vi "Read Bus.vi"(8 "error in (no error)":errorcluster, 11 "DigitalGraph.lvclass in":refnum<class "DigitalGraph.lvclass">) -> (0 "error out":errorcluster, 2 "Bus":refnum<vi>, 3 "DigitalGraph.lvclass out":refnum<class "DigitalGraph.lvclass">)   [LabVIEW 2015, in "DigitalGraph.lvclass"]
uses:
  DigitalGraph.lvclass
  DigitalGraph.lvclass/DigitalGraph.ctl
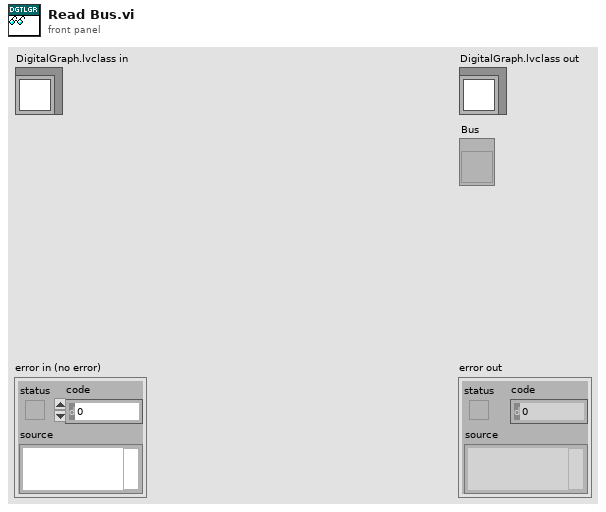
[diagram p1: front panel]
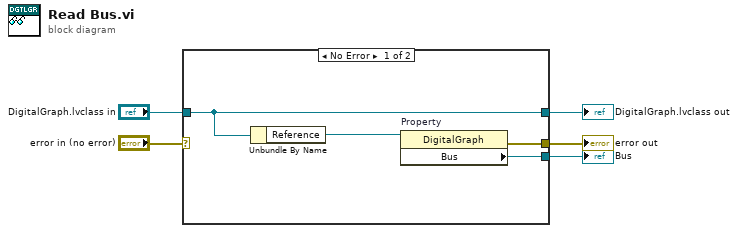
[diagram p0: block diagram]
diagram:
  n1 = case shown="No Error" "error in (no error)" {
    selector: "error in (no error)" -> [_ w11]
    tunnel: [w8 w11] -> w4
    tunnel: [w7 w10] -> w2
    tunnel: "DigitalGraph.lvclass in" -> [w7 w10]
    tunnel: [w9 _] -> w1
    frame No Error {
      n2 = Unbundle By Name(w7) -> ("Reference"=w6:refnum<vi>)
      n3 = property on="Property" class="DigitalGraph"(reference=w6) -> (error out=w8:errorcluster, "Bus"=w9:refnum<vi>)  [unwired: 1 in, 1 out]
    }
    frame Error {
    }
  }
  "error out" <- w4
  "DigitalGraph.lvclass out" <- w2
  "Bus" <- w1
